vi "SDK.vi"() -> ()   [LabVIEW 2015]
uses:
  C:/Users/mallman/Documents/git/SDKDlls/SDKNET/SDKNET/bin/Debug/SDKNET.dll
  SDKNET.dll
panel:
  in  "Array 2":string[](array[string])
  in  "Delete Objects":bool
  out "Array":dbl[][](array[numeric])
  in  "name":string="New Frame"
  in  "col":string="B"
  in  "Get Obj Transform":bool
  in  "name":string="New Frame"
  in  "col":string="B"
  in  "Transform":dbl[][](array[numeric])=[[1.0, 0.0, 0.0, 100.0], [0.0, 1.0, 0.0, 100.0], [0.0, 0.0, 1.0, 100.0], [0.0, 0.0, 0.0, 1.0]]
  in  "Construct Frame":bool
  in  "targ":string="fitPoint"
  in  "grp":string="BMain"
  in  "col":string="B"
  in  "Construct Point Fit To Points":bool
  out "GetActiveCollectionName":string
  in  "Get Active Col Name":bool
  in  "Delete Collection":bool
  out "MakePointNameRefListRuntimeSelect":string[](array[string])
  in  "nmDest":string
  in  "colDest":string
  in  "nmSrc":string
  in  "colSrc":string
  in  "Copy Object":bool
  in  "stop":bool
  in  "Get Pnt Ref List":bool
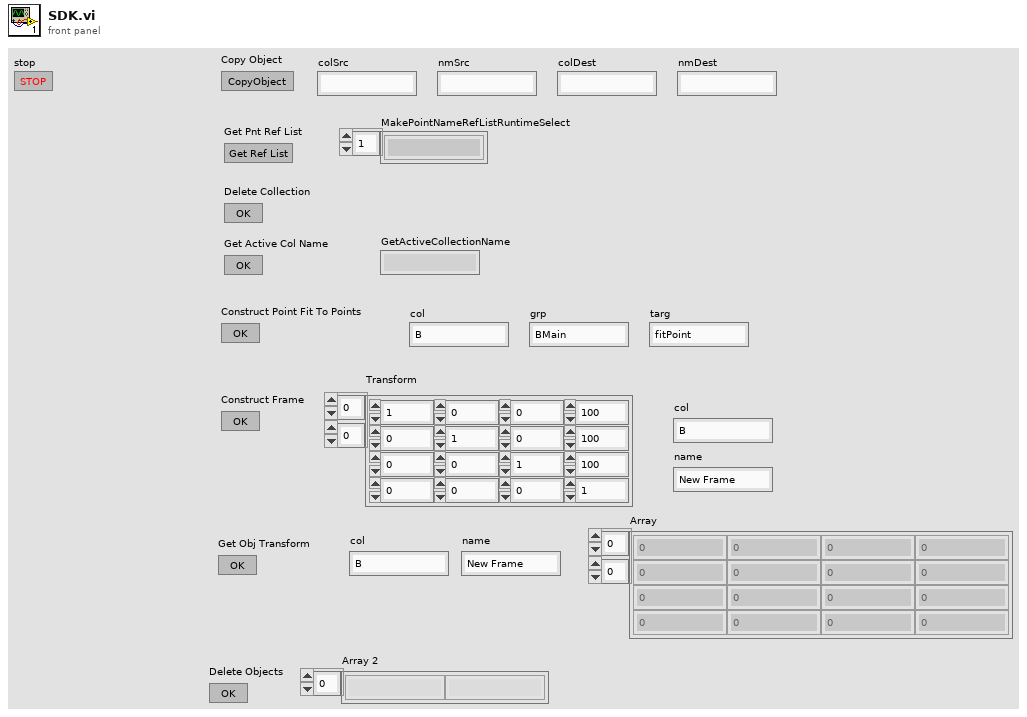
[diagram p1: front panel]
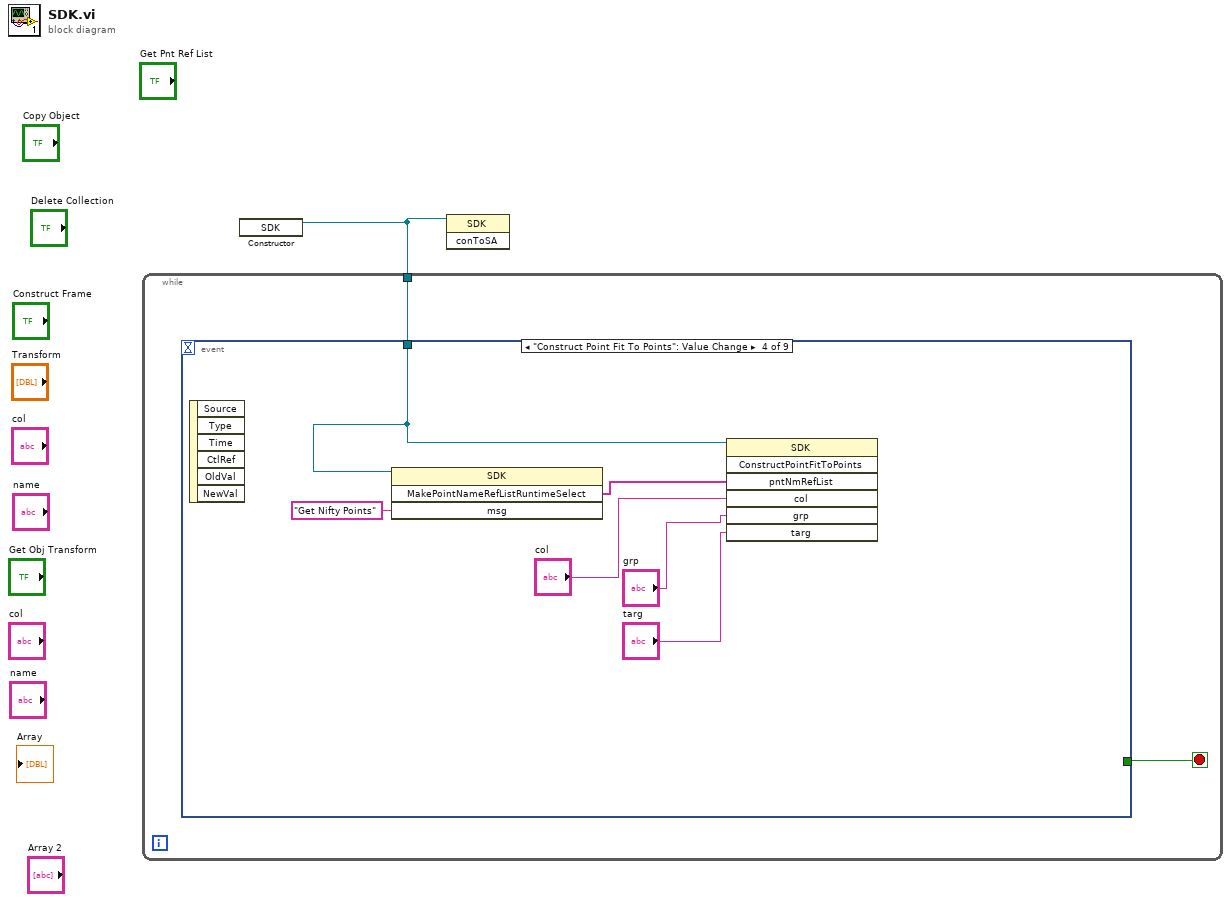
[diagram p0: block diagram]
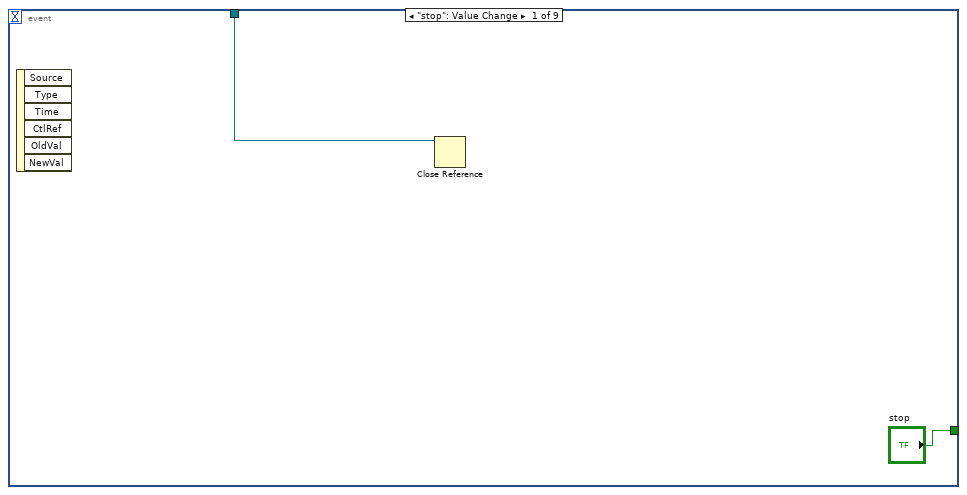
[diagram p2: hidden frame]
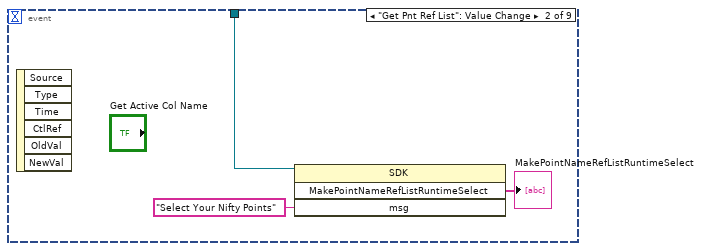
[diagram p3: hidden frame]
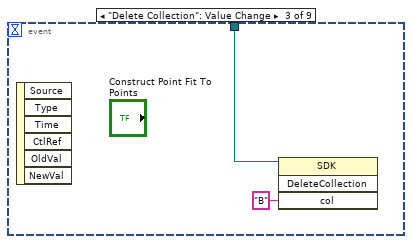
[diagram p4: hidden frame]
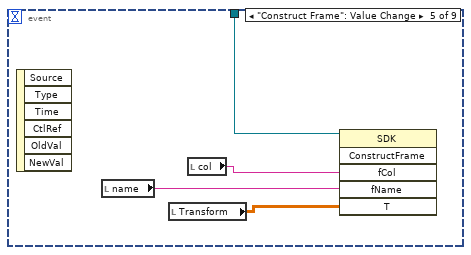
[diagram p5: hidden frame]
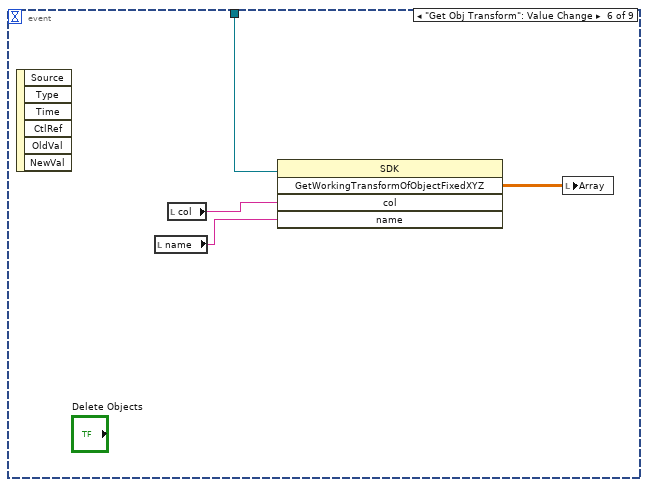
[diagram p6: hidden frame]
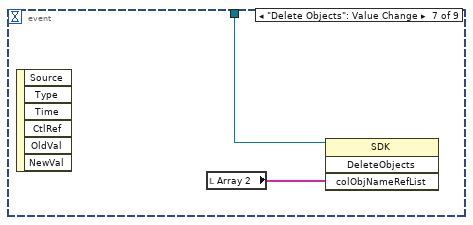
[diagram p7: hidden frame]
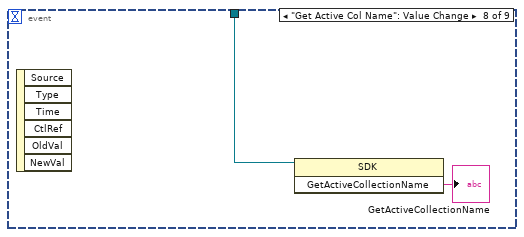
[diagram p8: hidden frame]
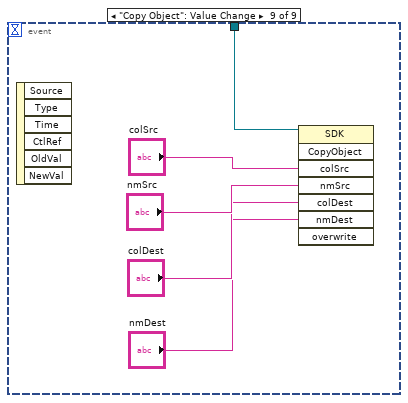
[diagram p9: hidden frame]
diagram:
  n1 = constructor class="SDK"() -> (reference out=w1:refnum<k24>)  [unwired: 3 in, 2 out]
  n2 = while {
    tunnel: w1 -> [w3]
    stop <- w2 stop-if-true
    n3 = event shown="[3] \"Construct Point Fit To Points\": Value Change" {
      selector: _ -> [_ _ _ _ _ _ _ _ _]
      dyn-events: _ -> [_ _ _ _ _ _ _ _ _]
      timeout: _ -> [_ _ _ _ _ _ _ _ _]
      tunnel: w3 -> [w4 w8 w10 w16 w20 w24 w26 w28 w33]
      tunnel: ["stop" _ _ _ _ _ _ _ _] -> w2
      event "stop": Value Change {
        n4 = event-data() -> ()  [unwired: 1 in, 6 out]
        n5 = Close Reference(reference=w4) -> ()  [unwired: 1 in, 1 out]
      }
      event "Get Pnt Ref List": Value Change {
        n6 = event-data() -> ()  [unwired: 1 in, 6 out]
        n7 = invoke class="SDK" method="MakePointNameRefListRuntimeSelect"(reference=w8, "msg"="Select Your Nifty Points") -> ("MakePointNameRefListRuntimeSelect"=→"MakePointNameRefListRuntimeSelect":string[])  [unwired: 2 in, 3 out]
      }
      event "Delete Collection": Value Change {
        n8 = event-data() -> ()  [unwired: 1 in, 6 out]
        n9 = invoke class="SDK" method="DeleteCollection"(reference=w10, "col"="B") -> ()  [unwired: 2 in, 4 out]
      }
      event "Construct Point Fit To Points": Value Change {
        n10 = event-data() -> ()  [unwired: 1 in, 6 out]
        n11 = invoke class="SDK" method="MakePointNameRefListRuntimeSelect"(reference=w16, "msg"="Get Nifty Points") -> ("MakePointNameRefListRuntimeSelect"=w15:string[])  [unwired: 2 in, 3 out]
        n12 = invoke class="SDK" method="ConstructPointFitToPoints"(reference=w16, "pntNmRefList"=w15, "col"="col", "grp"="grp", "targ"="targ") -> ()  [unwired: 2 in, 7 out]
      }
      event "Construct Frame": Value Change {
        n13 = event-data() -> ()  [unwired: 1 in, 6 out]
        n14 = local read "name"() -> (w17:string)
        n15 = local read "Transform"() -> (w19:dbl[][])
        n16 = local read "col"() -> (w18:string)
        n17 = invoke class="SDK" method="ConstructFrame"(reference=w20, "fCol"=w18, "fName"=w17, "T"=w19) -> ()  [unwired: 2 in, 6 out]
      }
      event "Get Obj Transform": Value Change {
        n18 = event-data() -> ()  [unwired: 1 in, 6 out]
        n19 = local read "name"() -> (w22:string)
        n20 = local read "col"() -> (w23:string)
        n21 = invoke class="SDK" method="GetWorkingTransformOfObjectFixedXYZ"(reference=w24, "col"=w23, "name"=w22) -> ("GetWorkingTransformOfObjectFixedXYZ"=w21:dbl[][])  [unwired: 2 in, 4 out]
        n22 = local write "Array"(w21) -> ()
      }
      event "Delete Objects": Value Change {
        n23 = event-data() -> ()  [unwired: 1 in, 6 out]
        n24 = local read "Array 2"() -> (w25:string[])
        n25 = invoke class="SDK" method="DeleteObjects"(reference=w26, "colObjNameRefList"=w25) -> ()  [unwired: 2 in, 4 out]
      }
      event "Get Active Col Name": Value Change {
        n26 = event-data() -> ()  [unwired: 1 in, 6 out]
        n27 = invoke class="SDK" method="GetActiveCollectionName"(reference=w28) -> ("GetActiveCollectionName"=→"GetActiveCollectionName":string)  [unwired: 2 in, 2 out]
      }
      event "Copy Object": Value Change {
        n28 = event-data() -> ()  [unwired: 1 in, 6 out]
        n29 = invoke class="SDK" method="CopyObject"(reference=w33, "colSrc"="colSrc", "nmSrc"="nmSrc", "colDest"="colDest", "nmDest"="nmDest") -> ()  [unwired: 3 in, 8 out]
      }
    }
  }
  n30 = invoke class="SDK" method="conToSA"(reference=w1) -> ()  [unwired: 2 in, 3 out]
